vi "TB-Globals.vi"() -> ()   [LabVIEW 2020]
panel:
  in  "Version":string="1.10"
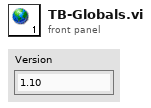
[diagram p1: front panel]
diagram:
